vi "RSZVB Set Frequency High Accuracy.vi"(8 "error in (no error)":errorcluster {"code" format="%.0x"}, 9 "High Accuracy (Off)":bool, 10 "Channel (1)":i32=1, 11 "VISA session":refnum<visa-resource-name>) -> (0 "error out":errorcluster {"code" format="%.0x"}, 3 "dup VISA session":refnum<visa-resource-name>)   [LabVIEW 2011]
doc: "This VI selects the mixer measurement with highest accuracy or with maximum speed.\n\nNote(s):\n\n(1) This VI can be used only with R&S ZVB instrument.\n\nRemote-control command(s):\n[SENSe<Ch>:]FREQuency:CONVersion:MIXer:HACCuracy ON | OFF"
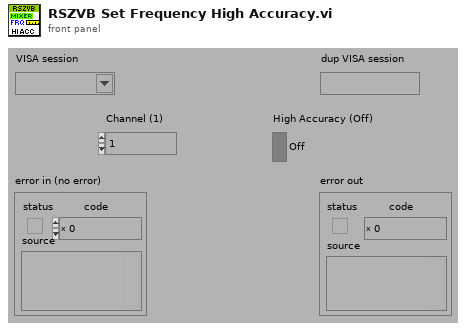
[diagram p1: front panel]
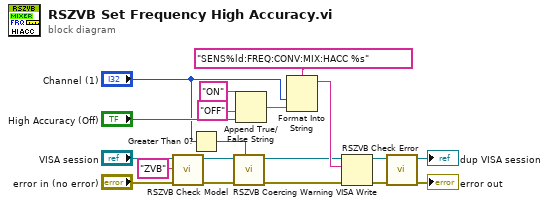
[diagram p0: block diagram]
diagram:
  n1 = call "RSZVB Check Model.vi"("error in (no error)"="error in (no error)", "Model"="ZVB", "VISA session"="VISA session") -> ("error out"=w3:errorcluster, "dup VISA session"=w4:refnum<visa-resource-name>)  [unwired: 7 in]
  n2 = Greater Than 0?(x="Channel (1)") -> (x > 0?=w8:bool)
  n3 = call "RSZVB Coercing Warning.vi"("In Range?"=w8, "error in (no error)"=w3, "VISA session"=w4) -> ("error out"=w11:errorcluster, "dup VISA session"=w12:refnum<visa-resource-name>)  [unwired: 7 in]
  n4 = Append True/False String(1:"High Accuracy (Off)", 2:"OFF" ("false string"), 3:"ON" ("true string")) -> (0:w16:string)  [unwired: 1 in]
  n5 = Format Into String(format string="SENS%ld:FREQ:CONV:MIX:HACC %s", "Channel (1)", w16) -> (resulting string=w17:string)  [unwired: 2 in, 1 out]
  n6 = VISA Write(VISA resource name=w12, write buffer=w17, error in (no error)=w11) -> (VISA resource name out=w19:refnum<visa-resource-name>, error out=w18:errorcluster)  [unwired: 1 out]
  n7 = call "RSZVB Check Error.vi"("error in (no error)"=w18, "VISA session"=w19) -> ("error out"=→"error out":errorcluster, "dup VISA session"=→"dup VISA session":refnum<visa-resource-name>)  [unwired: 8 in]
